vi "sync convert DBL seconds to sec and nsec.vi"(11 "seconds":dbl format="%#.6f") -> (2 "nsec":i64, 3 "sec":i64)   [LabVIEW 2013, in "Shared Memory runtime.lvclass"]
uses:
  Shared Memory runtime.lvclass
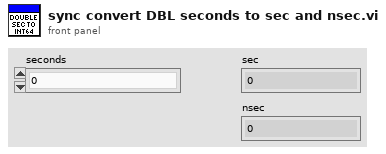
[diagram p1: front panel]
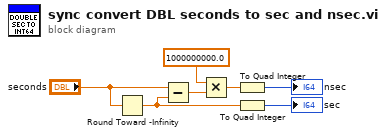
[diagram p0: block diagram]
diagram:
  n1 = Round Toward -Infinity(1:"seconds") -> (0:w3:dbl)
  n2 = Subtract(x="seconds", y=w3) -> (x-y=w5:dbl)
  n3 = Multiply(x=1000000000.0 ("y"), y=w5) -> (x*y=w6:dbl)
  n4 = To Quad Integer(1:w6) -> (0:→"nsec":i64)
  n5 = To Quad Integer(1:w3) -> (0:→"sec":i64)
